vi "Session Reservation with Session Factory.vi"(5 "service class":string, 7 "provided interface":string, 8 "error in":errorcluster, 10 "data in":T1, 11 "instrument type id":string="fake_instrument_type") -> (0 "error out":errorcluster, 2 "data out":T1, 3 "session reservation out":refnum<class "Session Reservation.lvclass">)   [LabVIEW 2020, in "Session Reservation Test Utilities.lvlib"]
uses:
  Session Reservation Test Utilities.lvlib
  Runtime/APIs/Session Management V1/Session Reservation/Data.ctl
  Runtime/APIs/Session Management V1/Connection Map/Connection Map.lvclass
  Runtime/APIs/Session Management V1/IReservation Observer/IReservation Observer.lvclass
  Runtime/APIs/Session Management V1/Session Reservation/Session and Driver Info.ctl
  Runtime/Sessions/Instrument Sessions/ISession Factory/ISession Factory.lvclass
  gRPC/Generated APIs/ni/measurementlink/sessionmanagement/v1/RPC Messages/ni_measurementlink_sessionmanagement_v1_SessionInformation.ctl
  gRPC/Generated APIs/ni/measurementlink/sessionmanagement/v1/RPC Messages/nidevice_grpc_Session.ctl
  gRPC/Generated APIs/ni/measurementlink/sessionmanagement/v1/RPC Messages/ni_measurementlink_sessionmanagement_v1_ChannelMapping.ctl
  Runtime/Sessions/Instrument Sessions/ISession Factory/Initialize and Close Session Behavior.ctl
  gRPC/Generated APIs/ni/measurementlink/sessionmanagement/v1/RPC Messages/ni_measurementlink_PinMapContext.ctl
  Runtime/APIs/Session Management V1/Session Reservation/Group Mapping.ctl
  Runtime/APIs/Session Management V1/Session Reservation/Session Reservation.lvclass
  Tests/Tests.Runtime/Measurement Server/Helpers/Fake Session Factory/Fake Session Factory.lvclass
  C:/dev/measurementlink-labview/Source/Runtime/Sessions/Instrument Sessions/ISession Factory/ISession Factory.lvclass
  gRPC/Generated APIs/ni/measurementlink/sessionmanagement/v1/ni.measurementlink.sessionmanagement.v1.api.lvlib
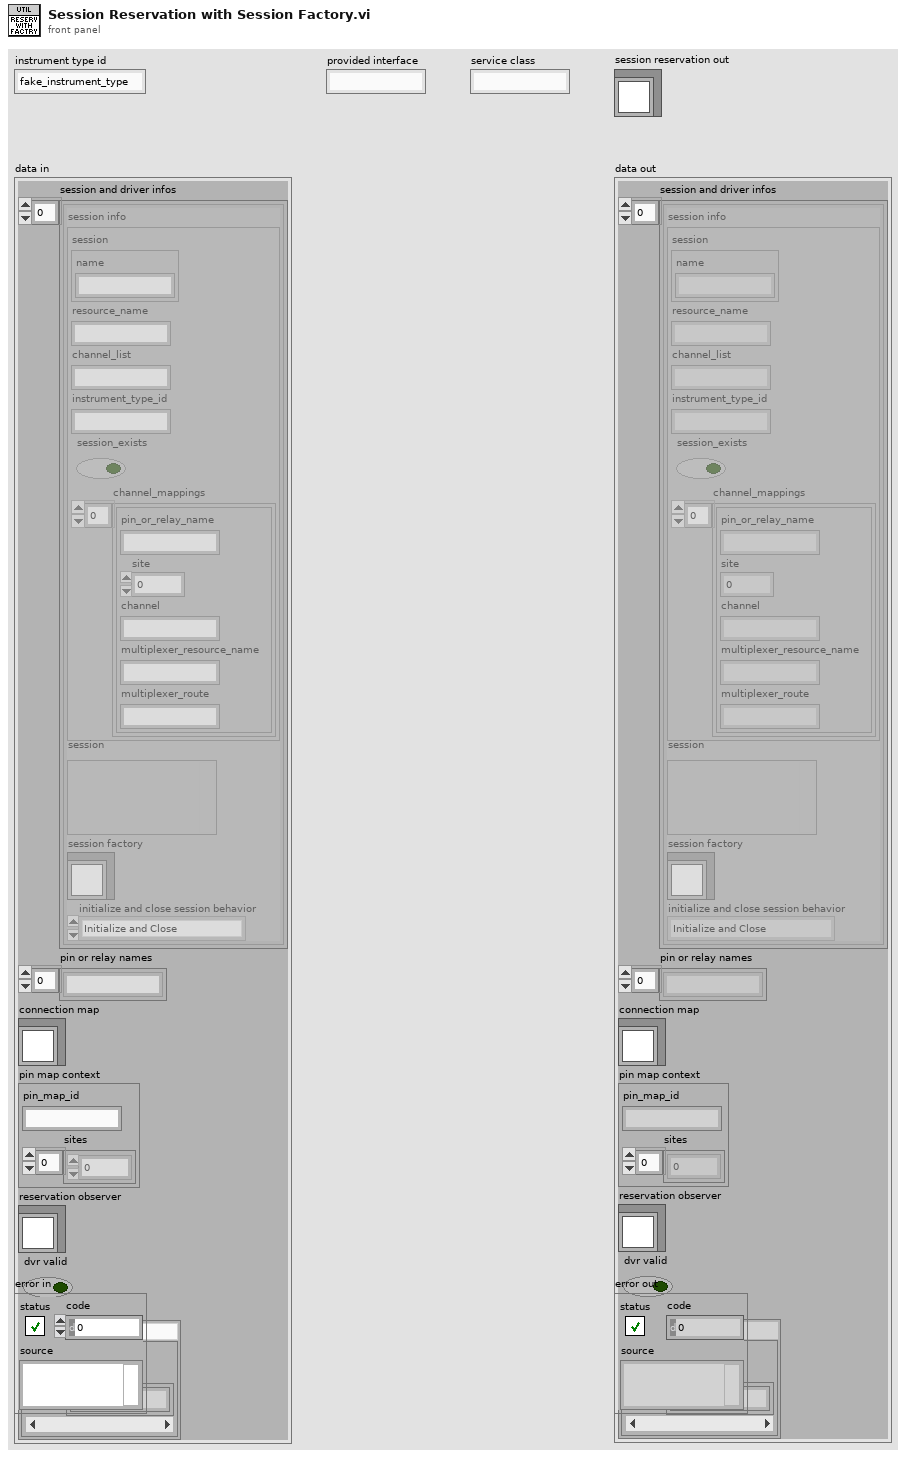
[diagram p1: front panel]
types:
  T1 = typedef "Plug-In SDK Session Management V1 API.lvlib/Session Reservation.lvclass/Data.ctl" = cluster{"session and driver infos":T2[], "pin or relay names":string[], "connection map":refnum<class "Connection Map.lvclass">, "pin map context":T7, "reservation observer":refnum<class "IReservation Observer.lvclass">, "dvr valid":bool, "group mappings":T8}
  T2 = typedef "Plug-In SDK Session Management V1 API.lvlib/Session Reservation.lvclass/Session and Driver Info.ctl" = cluster{"session info":T3, "session":variant, "session factory":refnum<class "ISession Factory.lvclass">, "initialize and close session behavior":T6}
  T3 = typedef "ni.measurementlink.sessionmanagement.v1.api.lvlib/ni_measurementlink_sessionmanagement_v1_SessionInformation.ctl" = cluster{"session":T4, "resource_name":string, "channel_list":string, "instrument_type_id":string, "session_exists":bool, "channel_mappings":T5[]}
  T4 = typedef "ni.measurementlink.sessionmanagement.v1.api.lvlib/nidevice_grpc_Session.ctl" = cluster{"name":string}
  T5 = typedef "ni.measurementlink.sessionmanagement.v1.api.lvlib/ni_measurementlink_sessionmanagement_v1_ChannelMapping.ctl" = cluster{"pin_or_relay_name":string, "site":i32, "channel":string, "multiplexer_resource_name":string, "multiplexer_route":string}
  T6 = typedef "Plug-In SDK Instrument Sessions.lvlib/ISession Factory.lvclass/Initialize and Close Session Behavior.ctl" = enum16{"Initialize and Close", "Attach and Detach", "Initialize and Detach", "Attach and Close"}
  T7 = typedef "ni.measurementlink.sessionmanagement.v1.api.lvlib/ni_measurementlink_PinMapContext.ctl" = cluster{"pin_map_id":string, "sites":i32[]}
  T8 = typedef "Plug-In SDK Session Management V1 API.lvlib/Session Reservation.lvclass/Group Mapping.ctl" = map{string, string[]}
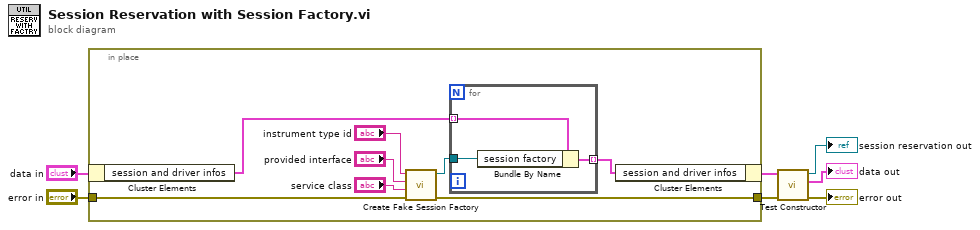
[diagram p0: block diagram]
diagram:
  n1 = in-place {
    in-place-border: "error in" -> [w15]
    in-place-border: [w11] -> w2
    n2 = in-place-cluster #1("data in") -> ("session and driver infos"=w14:T2[])
    n3 = call "Create Fake Session Factory.vi"("error in"=w15, "service class"="service class", "provided interface"="provided interface", "instrument type id"="instrument type id") -> ("error out"=w11:errorcluster, "fake session factory out"=w13:refnum<class "Fake Session Factory.lvclass">)  [unwired: 6 in]
    n4 = for {
      tunnel: w14 -> [w16] mode=indexing
      tunnel: w13 -> [w17]
      tunnel: [w18] -> w12 mode=indexing
      n5 = Bundle By Name(cluster=w16, "session factory"=w17) -> (w18:T2)
    }
    n6 = in-place-cluster #1("session and driver infos"=w12) -> (w1:T1)
  }
  n7 = call "Test Constructor.vi"("error in"=w2, "data in"=w1) -> ("error out"=→"error out":errorcluster, "data out"=→"data out":T1, "session reservation out"=→"session reservation out":refnum<class "Session Reservation.lvclass">)  [unwired: 7 in]
